vi "Measure_Decimate Dbl Array.vi"(7 "Leftover Last":dbl[](array[numeric]), 8 "Error":errorcluster, 9 "Factor":i32, 11 "DBL Array":dbl[](array[numeric])) -> (0 "Error Out":errorcluster, 3 "DBL Array Out":dbl[](array[numeric]), 5 "Leftover Out":dbl[](array[numeric]))   [LabVIEW 2025]
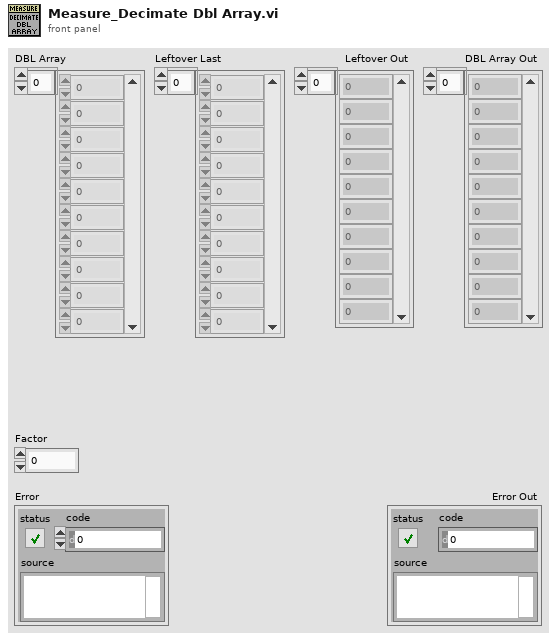
[diagram p1: front panel]
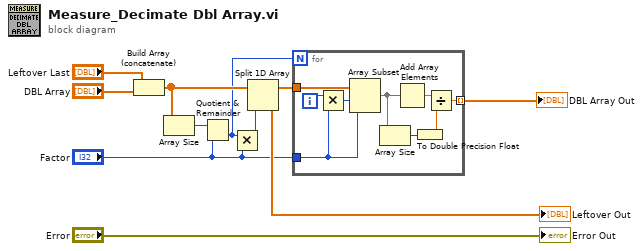
[diagram p0: block diagram]
diagram:
  n1 = Build Array (concatenate)("Leftover Last", "DBL Array") -> (w8:dbl[])
  n2 = Array Size(array=w8) -> (size(s)=w9:i32)
  n3 = Quotient & Remainder(x=w9, y="Factor") -> (floor(x/y)=w3:i32)  [unwired: 1 out]
  n4 = Multiply(x=w3, y="Factor") -> (x*y=w7:i32)
  n5 = Split 1D Array(array=w8, index=w7) -> (first subarray=w4:dbl[], second subarray=→"Leftover Out":dbl[])
  n6 = for {
    N: w3 -> [_]
    tunnel: w4 -> [w19]
    tunnel: "Factor" -> [w17]
    tunnel: [w12] -> w1 mode=indexing
    i -> [w20]
    n7 = Multiply(x=w20, y=w17) -> (x*y=w18:i32)
    n8 = Array Subset(array=w19, index=w18, length=w17) -> (w16:dbl[])
    n9 = Array Size(array=w16) -> (size(s)=w14:i32)
    n10 = Add Array Elements(numeric array=w16) -> (sum=w15:dbl)
    n11 = To Double Precision Float(number=w14) -> (double precision float=w13:dbl)
    n12 = Divide(x=w15, y=w13) -> (x/y=w12:dbl)
  }
  "DBL Array Out" <- w1
  "Error Out" <- "Error"
